vi "nested-array.vi"() -> ()   [LabVIEW 2025]
uses:
  <vilib>/numeric/Random Number (Range) U64.vi
  <vilib>/numeric/sub_Random U32.vi
panel:
  out "min value":i64
  out "max value":i64
  out "Array":i64[][](array[numeric])
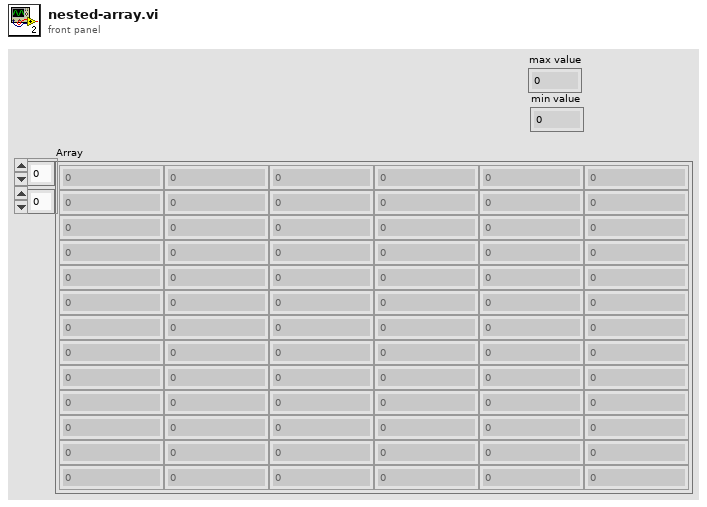
[diagram p1: front panel]
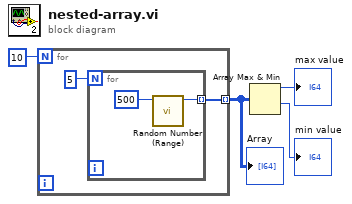
[diagram p0: block diagram]
diagram:
  n1 = for {
    N: 10 -> [_]
    tunnel: [w5] -> w3 mode=indexing
    n2 = for {
      N: 5 -> [_]
      tunnel: [w8] -> w5 mode=indexing
      n3 = call-poly <vilib>:"Random Number (Range).vi"("upper bound (100)"=u64 500) -> ("number"=w8:u64)  [unwired: 10 in]
    }
  }
  "Array" <- w3
  n4 = Array Max & Min(array=w3) -> (max value=→"max value":u64, min value=→"min value":u64)  [unwired: 2 out]
